vi "Clear State.vi"(8 "error in (no error)":errorcluster, 11 "Sync 2-Axis Stage Controller in":refnum<class "Sync 2-Axis Stage Controller.lvclass">) -> (0 "error out":errorcluster, 3 "Sync 2-Axis Stage Controller out":refnum<class "Sync 2-Axis Stage Controller.lvclass">)   [LabVIEW 2022 SP3, in "Sync 2-Axis Stage Controller.lvclass"]
uses:
  Sync 2-Axis Stage Controller.lvclass
  <vilib>/ErrorRing/Error Ring.xnode
  Sync 2-Axis Stage Controller.lvclass/Sync 2-Axis Stage Controller.ctl
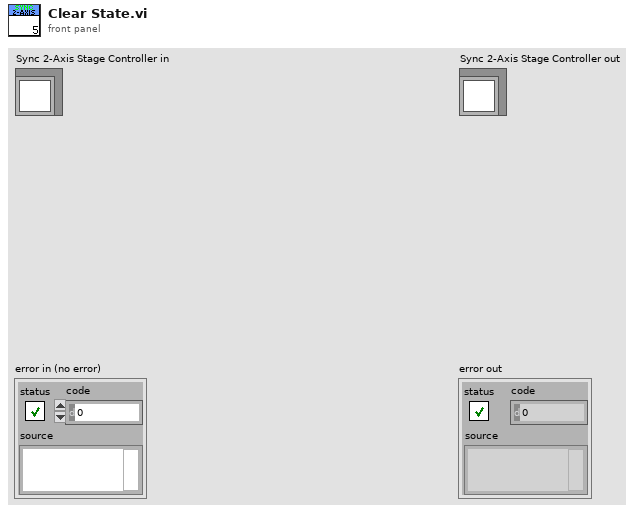
[diagram p1: front panel]
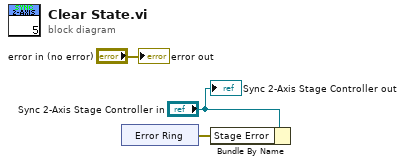
[diagram p0: block diagram]
diagram:
  n1 = xnode "Error Ring"() -> ("error out"=w2:errorcluster)
  n2 = Bundle By Name(cluster="Sync 2-Axis Stage Controller in", "Stage Error"=w2) -> ()  [unwired: 1 out]
  "error out" <- "error in (no error)"
  "Sync 2-Axis Stage Controller out" <- "Sync 2-Axis Stage Controller in"
